vi "Detect VISA communication port mMc.vi"(3 "error in (no error)":errorcluster) -> (5 "Port":T1={"P type"=1, "VISA resource name out"="", " Terminator"="\n\r", "Timeout"=300} {"Timeout" step=10; "P type" items=["none", "RS-232C", "IEEE-488.1", "IEEE-488.2"]}, 6 "Port OK":bool, 7 "Controller":string, 9 "error out":errorcluster)   [LabVIEW 2015]
doc: "检测VISA通信端口"
uses:
  <vilib>/Instr/_visa.llb/VISA Configure Serial Port (Instr).vi
panel:
  in  "STOP":bool
  in  "COM Port:":refnum<visa-resource-name>="COM4"
  out "P wt":bool
  in  "Controller address":i16=1
  out "msg":string="Start this application before turning on the\ncontroller or plugging in the USB cable"
  out "232 msg":string caption="Status log"
  in  "Baud":u16(ring)=5 caption="Baud rate" items=["1200", "2400", "4800", "9600", "19200", "38400", "57600", "115200"]
  in  "cont":bool
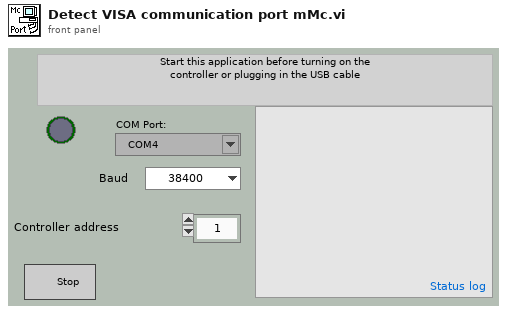
[diagram p1: front panel]
types:
  T1 = cluster{"P type":u16, "VISA resource name out":refnum<visa-resource-name>, " Terminator":string, "Timeout":i32}
  T2 = cluster{"milliseconds to wait":u32, "VISA resource name out":refnum<visa-resource-name>, string, "timeout":i32}
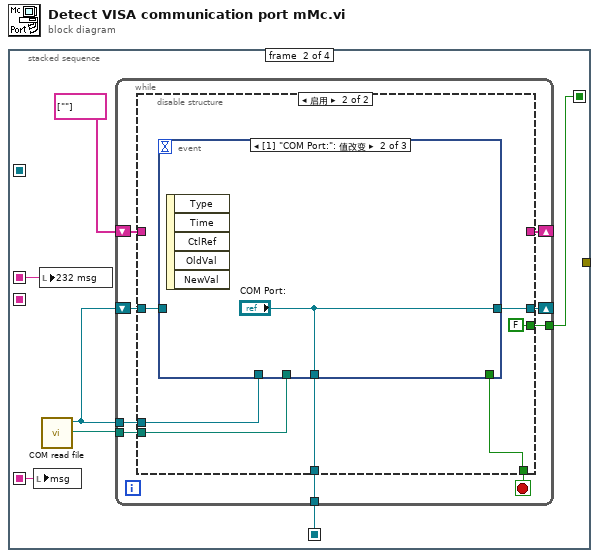
[diagram p0: block diagram]
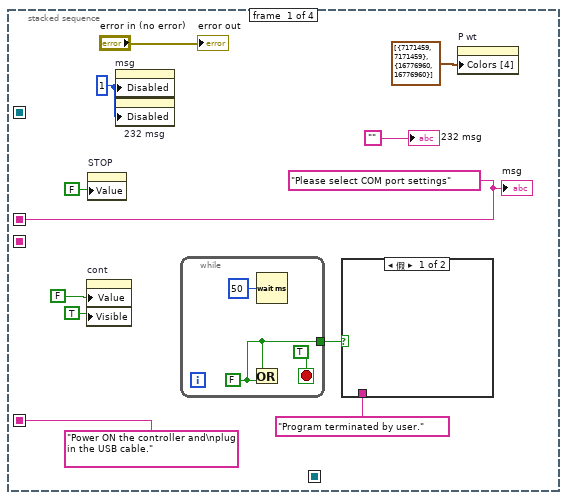
[diagram p2: hidden frame]
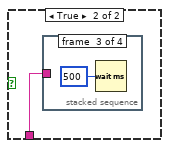
[diagram p3: hidden frame]
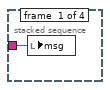
[diagram p4: hidden frame]
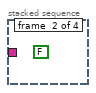
[diagram p5: hidden frame]
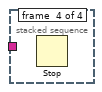
[diagram p6: hidden frame]
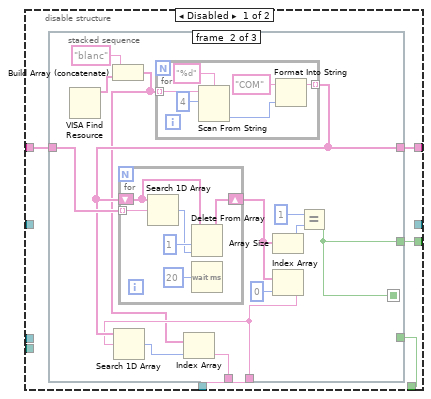
[diagram p7: hidden frame]
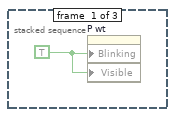
[diagram p8: hidden frame]
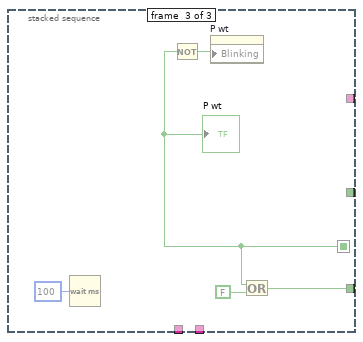
[diagram p9: hidden frame]
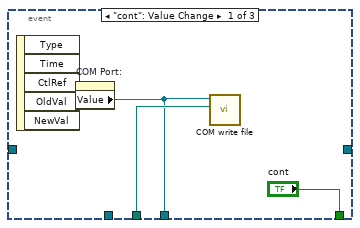
[diagram p10: hidden frame]
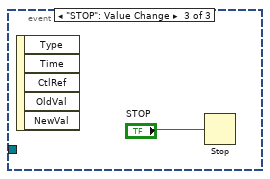
[diagram p11: hidden frame]
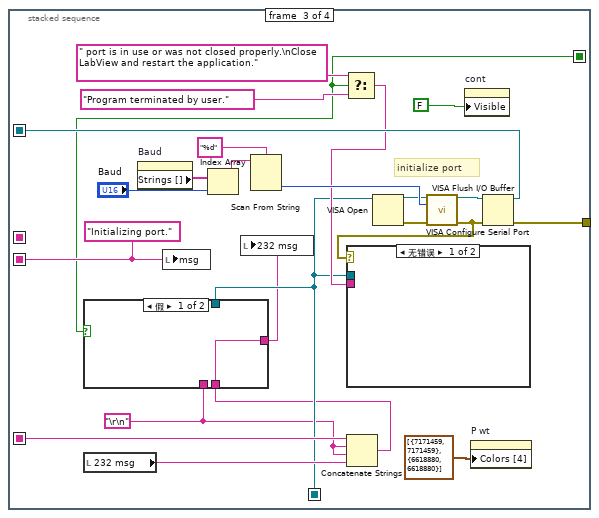
[diagram p12: hidden frame]
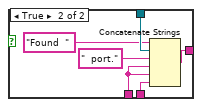
[diagram p13: hidden frame]
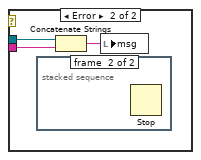
[diagram p14: hidden frame]
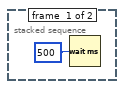
[diagram p15: hidden frame]
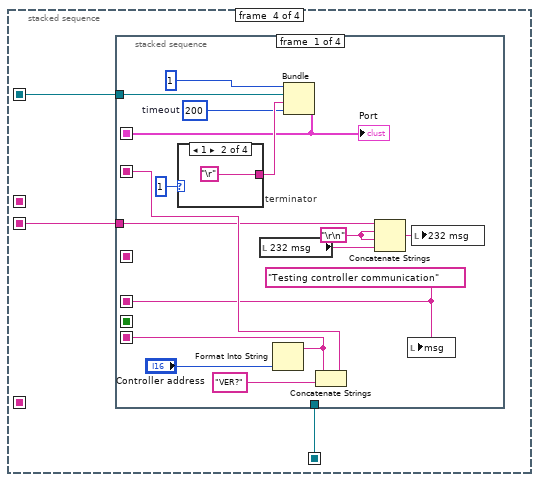
[diagram p16: hidden frame]
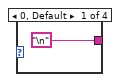
[diagram p17: hidden frame]
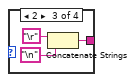
[diagram p18: hidden frame]
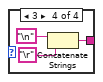
[diagram p19: hidden frame]
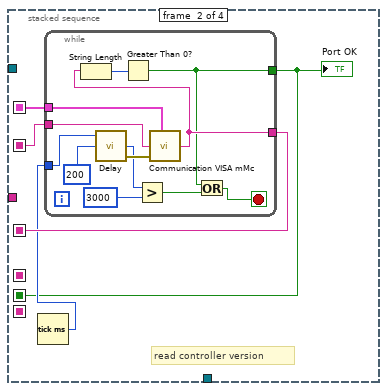
[diagram p20: hidden frame]
diagram:
  n1 = stacked-sequence {
    seq-local: [_ w23 _ _] -> [_ _ w87 w117]
    seq-local: [w8 _ _ _] -> [_ w22 _ _]
    seq-local: ["Power ON the controller and\nplug in the USB cable." ("232 msg") _ _ _] -> [_ w21 w104 _]
    seq-local: [_ _ w101 _] -> [_ _ _ w118]
    seq-local: [_ _ w93 _] -> [_ _ _ w119]
    seq-local: [_ w20 _ _] -> [_ _ w86 _]
    tunnel: [_ _ w82 _] -> _
    frame #0 {
      w8 = "Please select COM port settings" ("232 msg")
      w10 = u8 1 ("Write Attribute")
      n2 = property on="cont" class="Bool (严格)"("Value"=FALSE ("cont"), "Visible"=TRUE) -> ()  [unwired: 2 in, 2 out]
      n3 = property on="STOP" class="Bool (严格)"("Value"=FALSE ("STOP")) -> ()  [unwired: 2 in, 2 out]
      n4 = property on="msg" class="Str"("Disabled"=w10) -> ()  [unwired: 2 in, 2 out]
      n5 = property on="232 msg" class="Str"("Disabled"=w10) -> ()  [unwired: 2 in, 2 out]
      n6 = while {
        tunnel: [w15] -> w5
        stop <- TRUE stop-if-true
        w15 = FALSE ("y")
        n7 = Or(x=w15, y=w15) -> ()  [unwired: 1 out]
        n8 = Wait (ms)(milliseconds to wait=u32 50) -> ()  [unwired: 1 out]
      }
      n9 = case shown="假" w5 {
        tunnel: "Program terminated by user." -> [_ w12]
        frame False {
        }
        frame True {
          n10 = stacked-sequence {
            tunnel: w12 -> [w13 _ _ _]
            frame #0 {
              n11 = local write "msg"(w13) -> ()
            }
            frame #1 {
              (unwired) FALSE ("exit")
            }
            frame #2 {
              n12 = Wait (ms)(milliseconds to wait=u32 500) -> ()  [unwired: 1 out]
            }
            frame #3 {
              n13 = Stop() -> ()  [unwired: 1 in]
            }
          }
        }
      }
      n14 = property on="P wt" class="Bool (严格)"("Colors [4]"=cluster{u32, u32}[] [{7171459, 7171459}, {16776960, 16776960}]) -> ()  [unwired: 2 in, 2 out]
      "msg" <- w8
      "error out" <- "error in (no error)"
      "232 msg" <- ""
    }
    frame #1 {
      n15 = local write "msg"(w21) -> ()
      n16 = local write "232 msg"(w22) -> ()
      n17 = call <instrlib>:"COM read file.vi"() -> ("COM file path"=w19:path, "COM port"=w18:refnum<visa-resource-name>)  [unwired: 10 in]
      n18 = while {
        shift-right: [w32] -> _
        shift-left: string[] [""] -> [w33]
        tunnel: [w31] -> w23
        tunnel: [w29] -> w20
        shift-right: [w26] -> _
        shift-left: w18 -> [w28]
        tunnel: w19 -> [w27]
        tunnel: w18 -> [w25]
        stop <- w30 stop-if-true
        n19 = disable-structure shown="启用" {
          disable-tunnel: w33 -> [w38 _]
          disable-tunnel: [w37 _] -> w32
          disable-tunnel: [w36 w75] -> w31
          disable-tunnel: [w35 w76] -> w30
          disable-tunnel: [w34 FALSE] -> w29
          disable-tunnel: w25 -> [_ w74]
          disable-tunnel: [_ w73] -> w26
          disable-tunnel: w28 -> [_ w72]
          disable-tunnel: w27 -> [_ w71]
          frame Disabled {
            n20 = stacked-sequence {
              seq-local: [_ w40 _] -> [_ _ w66]
              tunnel: w38 -> [_ w52 _]
              tunnel: [_ w49 _] -> w37
              tunnel: [_ w45 _] -> _
              tunnel: [_ w44 _] -> w36
              tunnel: [_ _ w67] -> w35
              tunnel: [_ w40 _] -> w34
              frame #0 {
                w39 = TRUE
                n21 = property on="P wt" class="Bool (严格)"("Blinking"=w39, "Visible"=w39) -> ()  [unwired: 2 in, 2 out]
              }
              frame #1 {
                n22 = VISA Find Resource() -> (3:w43:string[])  [unwired: 3 in, 2 out]
                n23 = Build Array (concatenate)("blanc", w43) -> (w42:string[])
                n24 = for {
                  tunnel: w42 -> [w63] mode=indexing
                  tunnel: [w60] -> w49 mode=indexing
                  n25 = Scan From String(format string="%d", input string=w63, initial scan location=u32 4) -> (output 1=w62:i32)  [unwired: 2 in, 3 out]
                  n26 = Format Into String(initial string="COM", w62) -> (resulting string=w60:string)  [unwired: 2 in, 1 out]
                }
                n27 = for {
                  shift-right: [w55] -> w48
                  shift-left: w49 -> [w56]
                  tunnel: w52 -> [w58] mode=indexing
                  n28 = Search 1D Array(1D array=w56, element=w58) -> (index of element=w54:i32)  [unwired: 1 in]
                  n29 = Delete From Array(array=w56, length=1, index=w54) -> (array with subset deleted=w55:string[])  [unwired: 1 out]
                  n30 = Wait (ms)(milliseconds to wait=u32 20) -> ()  [unwired: 1 out]
                }
                n31 = Array Size(array=w48) -> (size(s)=w51:i32)
                n32 = Index Array(array=w48, index=0) -> (element=w44:string)
                n33 = Search 1D Array(1D array=w49, element=w44) -> (index of element=w46:i32)  [unwired: 1 in]
                n34 = Index Array(array=w42, index=w46) -> (element=w45:string)
                n35 = Equal?(x=1, y=w51) -> (x = y?=w40:bool)
              }
              frame #2 {
                n36 = Wait (ms)(milliseconds to wait=u32 100) -> ()  [unwired: 1 out]
                n37 = Not(x=w66) -> (.not. x?=w69:bool)
                n38 = property on="P wt" class="Bool (严格)"("Blinking"=w69) -> ()  [unwired: 2 in, 2 out]
                n39 = Or(x=w66, y=FALSE) -> (x .or. y?=w67:bool)
                "P wt" <- w66
              }
            }
          }
          frame Enabled {
            n40 = event shown="[1] \"COM Port:\": 值改变" {
              selector: _ -> [_ _ _]
              dyn-events: _ -> [_ _ _]
              timeout: _ -> [_ _ _]
              tunnel: ["cont" _ _] -> w76
              tunnel: [w77 "COM Port:" _] -> w75
              tunnel: w74 -> [_ _ _]
              tunnel: [_ "COM Port:" _] -> w73
              tunnel: w72 -> [_ _ _]
              tunnel: w71 -> [w78 _ _]
              event "cont": Value Change {
                n41 = event-data() -> ()  [unwired: 1 in, 5 out]
                n42 = property on="COM Port:" class="VISAName"() -> ("Value"=w77:refnum<visa-resource-name>)  [unwired: 2 in, 2 out]
                n43 = call <instrlib>:"COM write file.vi"("COM file path"=w78, "COM Port:"=w77) -> ()  [unwired: 10 in]
              }
              event "COM Port:": Value Change {
                n44 = event-data() -> ()  [unwired: 1 in, 5 out]
              }
              event "STOP": Value Change {
                n45 = event-data() -> ()  [unwired: 1 in, 5 out]
                n46 = Stop(stop? (T)="STOP") -> ()
              }
            }
          }
        }
      }
    }
    frame #2 {
      w101 = "Initializing port."
      w84 = "\r\n"
      # "initialize port"
      n47 = local read "232 msg"() -> (w103:string)
      n48 = property on="Baud" class="Ring (严格)"() -> ("Strings []"=w100:string[])  [unwired: 2 in, 2 out]
      n49 = local write "msg"(w101) -> ()
      n50 = Index Array(array=w100, index="Baud") -> (element=w99:string)
      n51 = Scan From String(format string="%d" ("Format String"), input string=w99) -> (output 1=w96:i32)  [unwired: 3 in, 3 out]
      n52 = Select(t=" port is in use or was not closed properly.\nClose LabView and restart the application.", s=w86, f="Program terminated by user.") -> (s? t:f=w88:string)
      n53 = Concatenate Strings(w104, w84, w84, w103) -> (w83:string)
      n54 = case shown="假" w86 {
        tunnel: w87 -> [_ w112]
        tunnel: [w106 w109] -> w85
        tunnel: w84 -> [_ w108]
        tunnel: w83 -> [w106 w107]
        frame False {
        }
        frame True {
          n55 = Concatenate Strings("Found  " ("string"), w112, "  port." ("string"), w108, w108, w107) -> (w109:string)
        }
      }
      n56 = local write "232 msg"(w85) -> ()
      n57 = VISA Open(VISA resource name=w87) -> (VISA resource name=w92:refnum<visa-resource-name>, error out=w97:errorcluster)  [unwired: 4 in]
      n58 = call-poly "VISA Configure Serial Port"("VISA resource name"=w92, "baud rate (9600)"=w96, "error in (no error)"=w97) -> ("VISA resource name out"=w95:refnum<visa-resource-name>, "error out"=w91:errorcluster)  [unwired: 11 in]
      n59 = case shown="无错误" w91 {
        tunnel: w87 -> [_ w114]
        tunnel: w88 -> [_ w113]
        frame No Error {
        }
        frame Error {
          n60 = stacked-sequence {
            frame #0 {
              n61 = Wait (ms)(milliseconds to wait=u32 500) -> ()  [unwired: 1 out]
            }
            frame #1 {
              n62 = Stop() -> ()  [unwired: 1 in]
            }
          }
          n63 = Concatenate Strings(w114, w113) -> (w115:string)
          n64 = local write "msg"(w115) -> ()
        }
      }
      n65 = property on="cont" class="Bool (严格)"("Visible"=FALSE) -> ()  [unwired: 2 in, 2 out]
      n66 = property on="P wt" class="Bool (严格)"("Colors [4]"=cluster{u32, u32}[] [{7171459, 7171459}, {6618880, 6618880}]) -> ()  [unwired: 2 in, 2 out]
      n67 = VISA Flush I/O Buffer(VISA resource name=w95, error in (no error)=w91) -> (VISA resource name out=w93:refnum<visa-resource-name>, error out=w82:errorcluster)  [unwired: 1 in]
    }
    frame #3 {
      n68 = stacked-sequence {
        seq-local: [w120 _ _ _] -> [_ w147 _ _]
        seq-local: [_ w143 _ _] -> [_ _ w168 _]
        seq-local: [_ w145 _ _] -> [_ _ w165 _]
        seq-local: [w131 _ _ _] -> [_ w146 _ _]
        seq-local: [w130 _ _ _] -> [_ _ w164 _]
        seq-local: [w121 _ _ _] -> [_ _ w160 _]
        tunnel: w119 -> [w123 _ w167 _]
        tunnel: w118 -> [w122 _ _ _]
        tunnel: w117 -> [_ _ w166 _]
        frame #0 {
          w125 = "\r\n"
          w121 = "Testing controller communication"
          w133 = 200  # timeout
          n69 = case "terminator" shown="1" u32 1 ("milliseconds to wait") {
            tunnel: ["\n" "\r" w137 w140] -> w134
            frame 0, Default {
            }
            frame 1 {
            }
            frame 2 {
              n70 = Concatenate Strings ("terminator")("\r", "\n") -> (w137:string)
            }
            frame 3 {
              n71 = Concatenate Strings ("terminator")("\n", "\r") -> (w140:string)
            }
          }
          n72 = local read "232 msg"() -> (w124:string)
          n73 = Format Into String("Controller address") -> (resulting string=w130:string)  [unwired: 3 in, 1 out]
          n74 = Bundle("milliseconds to wait"=u32 1, "VISA resource name out"=w123, w134, "timeout"=w133) -> (w120:T2)  [unwired: 1 in]
          "Port" <- w120
          n75 = Concatenate Strings ("terminator")(w130, "VER?" ("Command")) -> (w131:string)
          n76 = Concatenate Strings(w122, w125, w125, w124) -> (w126:string)
          n77 = local write "msg"(w121) -> ()
          n78 = local write "232 msg"(w126) -> ()
        }
        frame #1 {
          # "read controller version"
          n79 = Tick Count (ms)() -> (millisecond timer value=w144:u32)
          n80 = while {
            tunnel: w147 -> [w159]
            tunnel: w146 -> [w155]
            tunnel: [w158] -> w145
            tunnel: [w148] -> w143
            tunnel: w144 -> [w154]
            stop <- w150 stop-if-true
            n81 = call <instrlib>:"Delay.vi"("old timer value"=w154, "milliseconds to wait"=200) -> ("elapsed time"=w152:u32, "error out"=w156:errorcluster)  [unwired: 5 in, 1 out]
            n82 = Greater?(x=w152, y=3000) -> (0:w149:bool)
            n83 = call <instrlib>:"Communication VISA mMc.vi"("Port"=w159, "Command"=w155, "error in (no error)"=w156) -> ("Return"=w158:string)  [unwired: 3 in, 3 out]
            n84 = String Length(string=w158) -> (length=w157:i32)
            n85 = Greater Than 0?(x=w157) -> (x > 0?=w148:bool)
            n86 = Or(x=w148, y=w149) -> (x .or. y?=w150:bool)
          }
          "Port OK" <- w143
        }
        frame #2 {
          w162 = "\r\n"
          n87 = local read "232 msg"() -> (w161:string)
          n88 = case shown="真" w168 {
            tunnel: w167 -> [w169 _]
            tunnel: w166 -> [_ w172]
            tunnel: w165 -> [_ w174]
            tunnel: w164 -> [_ w171]
            frame False {
              n89 = VISA Close(VISA resource name=w169) -> ()  [unwired: 1 in, 1 out]
              n90 = local write "msg"("Controller did not respond to a VER? command.\nMake sure the addrss and the Baud rate are correct." ("msg")) -> ()
            }
            frame True {
              n91 = Concatenate Strings("Found controller # " ("msg"), w171, " on port " ("msg"), w172, "\r\n", w174) -> (w176:string)
              n92 = local write "msg"(w176) -> ()
              "Controller" <- w172
            }
          }
          n93 = Concatenate Strings(w160, w162, w162, w161) -> (w163:string)
          n94 = local write "232 msg"(w163) -> ()
        }
        frame #3 {
          n95 = Wait (ms)(milliseconds to wait=u32 1000) -> ()  [unwired: 1 out]
        }
      }
    }
  }
